vi "FindDivDigitTwoBy.vi"(0 "Normalized A":T1, 1 "premultiplied array":cluster{"A":T1, "stop":bool}[](array[cluster]), 2 "Denom Info":cluster{"Denom":i32, "Offset":i32}) -> (3 "A Copy":T1, 4 "Exact Divide":bool, 5 "Digit":i32, 6 "premultiplied array out":cluster{"A":T1, "stop":bool}[](array[cluster]))   [LabVIEW 2025]
uses:
  Number.ctl
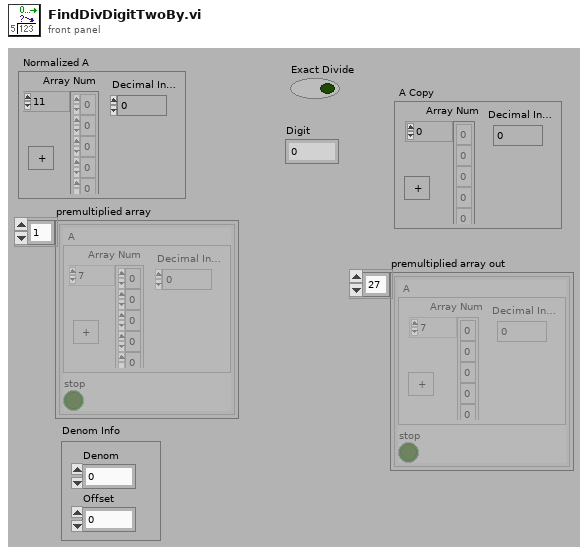
[diagram p1: front panel]
types:
  T1 = typedef "Number.ctl" = cluster{"Array Num":i8[], "Decimal Index":i32, "stop":bool}
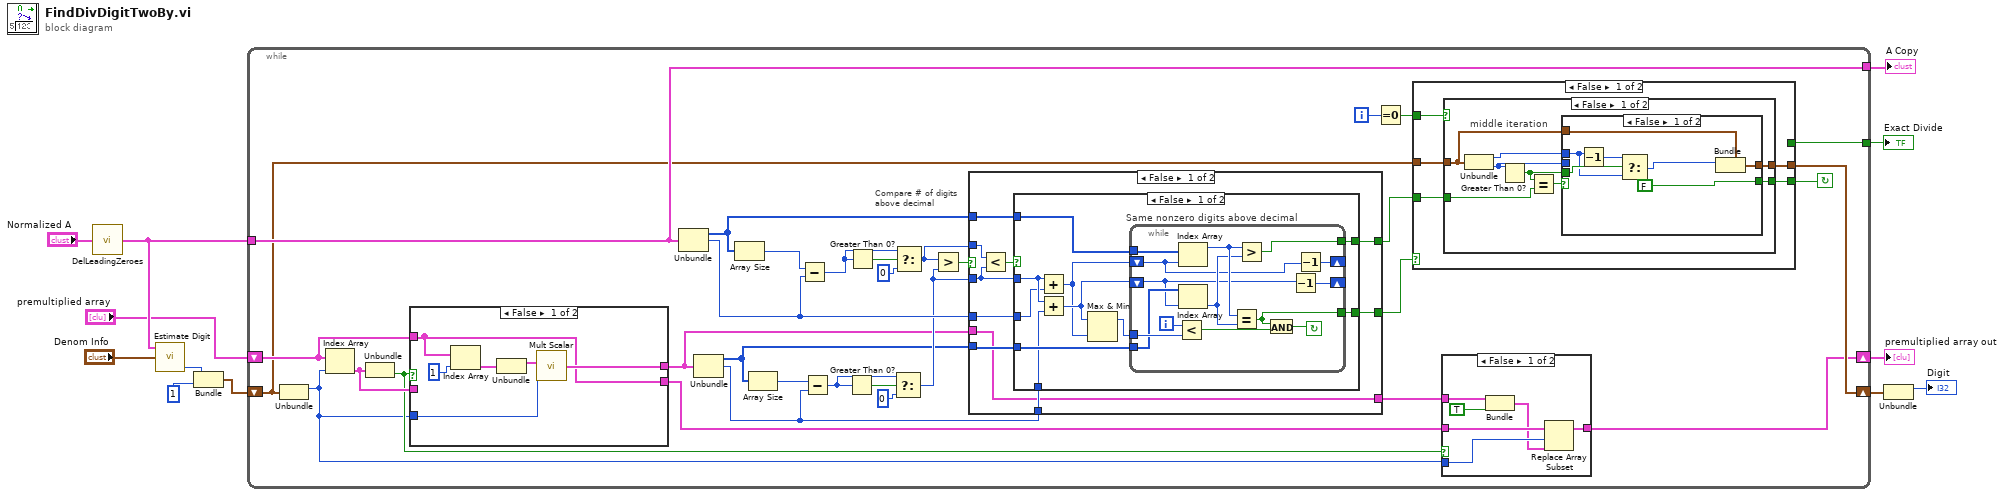
[diagram p0: block diagram]
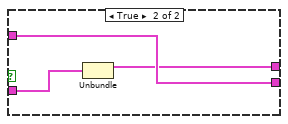
[diagram p3: hidden frame]
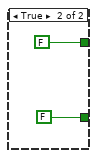
[diagram p4: hidden frame]
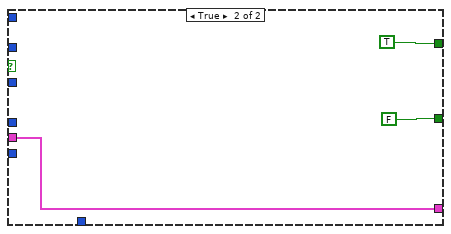
[diagram p5: hidden frame]
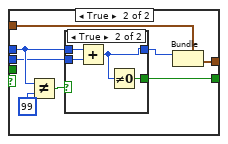
[diagram p6: hidden frame]
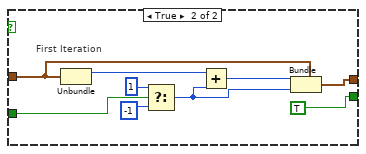
[diagram p8: hidden frame]
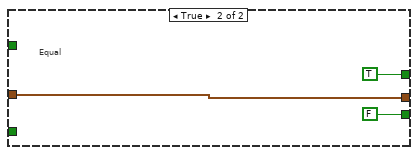
[diagram p9: hidden frame]
diagram:
  n1 = call "DelLeadingZeroes.vi"("A 2"="Normalized A") -> ("A"=w6:T1)
  n2 = call "Estimate Digit.vi"("Denom Info"="Denom Info", "A"=w6) -> ("Estimated Digit"=w5:i32)  [unwired: 3 in]
  n3 = Bundle("Estimated Digit"=w5, 1) -> (w3:cluster{"Estimated Digit":i32, i32})  [unwired: 1 in]
  n4 = while {
    tunnel: w6 -> [w24]
    shift-right: [w44] -> w10
    shift-left: w3 -> [w22]
    tunnel: [w42] -> w12
    tunnel: [w24] -> w8
    shift-right: [w19] -> w7
    shift-left: "premultiplied array" -> [w23]
    i -> [w13]
    stop <- w43 continue-if-true
    # "Compare # of digits above decimal"
    n5 = Unbundle(w22) -> ("Estimated Digit"=w17:i32)  [unwired: 1 out]
    n6 = Index Array(array=w23, index=w17) -> (element=w21:cluster{"A":T1, "stop":bool})
    n7 = Unbundle(w21) -> ("stop"=w18:bool)  [unwired: 1 out]
    n8 = case shown="False" w18 {
      tunnel: [w55 w58] -> w16
      tunnel: w17 -> [w57 _]
      tunnel: w23 -> [w52 w60]
      tunnel: [w52 w60] -> w20
      tunnel: w21 -> [_ w59]
      frame False {
        n9 = Index Array(array=w52, index=1 ("f")) -> (element=w53:cluster{"A":T1, "stop":bool})
        n10 = Unbundle(w53) -> ("A"=w56:T1)  [unwired: 1 out]
        n11 = call "Mult Scalar.vi"("A"=w56, "Scalar"=w57) -> ("A x Scalar"=w55:T1)  [unwired: 3 in]
      }
      frame True {
        n12 = Unbundle(w59) -> ("A"=w58:T1)  [unwired: 1 out]
      }
    }
    n13 = Unbundle(w24) -> ("Array Num"=w27:i8[], "Decimal Index"=w40:i32)  [unwired: 1 out]
    n14 = Unbundle(w16) -> ("Array Num"=w29:i8[], "Decimal Index"=w39:i32)  [unwired: 1 out]
    n15 = Array Size(array=w27) -> (size(s)=w28:i32)
    n16 = Array Size(array=w29) -> (size(s)=w30:i32)
    n17 = Subtract(x=w28, y=w40) -> (x-y=w32:i32)
    n18 = Subtract(x=w30, y=w39) -> (x-y=w31:i32)
    n19 = Greater Than 0?(x=w31) -> (x > 0?=w35:bool)
    n20 = Greater Than 0?(x=w32) -> (x > 0?=w36:bool)
    n21 = Select(t=w31, s=w35, f=0) -> (s? t:f=w33:i32)
    n22 = Select(t=w32, s=w36, f=0) -> (s? t:f=w37:i32)
    n23 = Greater?(x=w37, y=w33) -> (0:w41:bool)
    n24 = case shown="False" w41 {
      tunnel: [w69 TRUE] -> w26
      tunnel: w29 -> [w68 _]
      tunnel: w33 -> [w63 _]
      tunnel: w37 -> [w62 _]
      tunnel: w27 -> [w67 _]
      tunnel: [w66 FALSE] -> w25
      tunnel: w40 -> [w65 _]
      tunnel: w39 -> [w64 _]
      tunnel: w16 -> [w61 w97]
      tunnel: [w61 w97] -> w15
      frame False {
        n25 = Less?(x=w62, y=w63) -> (x < y?=w70:bool)
        n26 = case shown="False" w70 {
          tunnel: [w78 FALSE] -> w69
          tunnel: w68 -> [w79 _]
          tunnel: w67 -> [w80 _]
          tunnel: [w74 FALSE] -> w66
          tunnel: w65 -> [w76 _]
          tunnel: w64 -> [w75 _]
          tunnel: w63 -> [w77 _]
          frame False {
            # "Same nonzero digits above decimal"
            n27 = Add(x=w77, y=w76) -> (x+y=w71:i32)
            n28 = Add(x=w77, y=w75) -> (x+y=w72:i32)
            n29 = Max & Min(x=w72, y=w71) -> (max(x,y)=w73:i32)  [unwired: 1 out]
            n30 = while {
              tunnel: w73 -> [w88]
              tunnel: [w89] -> w74
              tunnel: [w90] -> w78
              tunnel: w79 -> [w85]
              tunnel: w80 -> [w86]
              shift-right: [w83] -> _
              shift-left: w71 -> [w81]
              shift-right: [w84] -> _
              shift-left: w72 -> [w82]
              i -> [w87]
              stop <- w93 continue-if-true
              n31 = Less?(x=w87, y=w88) -> (x < y?=w94:bool)
              n32 = Index Array(array=w86, index=w81) -> (element=w92:i8)
              n33 = Index Array(array=w85, index=w82) -> (element=w91:i8)
              n34 = Equal?(x=w92, y=w91) -> (x = y?=w89:bool)
              n35 = Greater?(x=w92, y=w91) -> (0:w90:bool)
              n36 = And(x=w89, y=w94) -> (x .and. y?=w93:bool)
              n37 = Decrement(x=w82) -> (x-1=w84:i32)
              n38 = Decrement(x=w81) -> (x-1=w83:i32)
            }
          }
          frame True {
          }
        }
      }
      frame True {
      }
    }
    n39 = Equal To 0?(x=w13) -> (x = 0?=w14:bool)
    n40 = case shown="False" w25 {
      tunnel: w22 -> [w102 w145]
      tunnel: w26 -> [w103 _]
      tunnel: w14 -> [w104 _]
      tunnel: [w101 w145] -> w44
      tunnel: [w100 FALSE] -> w43
      tunnel: [_ TRUE] -> w42
      frame False {
        n41 = case shown="False" w104 {
          tunnel: w103 -> [w112 w142]
          tunnel: w102 -> [w106 w137]
          tunnel: [w109 w135] -> w101
          tunnel: [w110 TRUE] -> w100
          frame False {
            # "middle iteration"
            n42 = Unbundle(w106) -> ("Estimated Digit"=w107:i32, w108:i32)
            n43 = Greater Than 0?(x=w108) -> (x > 0?=w105:bool)
            n44 = Equal?(x=w105, y=w112) -> (x = y?=w111:bool)
            n45 = case shown="False" w111 {
              tunnel: [FALSE w120] -> w110
              tunnel: [w115 w127] -> w109
              tunnel: w108 -> [_ w122]
              tunnel: w107 -> [w117 w123]
              tunnel: w106 -> [w113 w126]
              tunnel: w105 -> [w118 _]
              frame False {
                n46 = Decrement(x=w117) -> (x-1=w116:i32)
                n47 = Select(t=w116, s=w118, f=w117) -> (s? t:f=w114:i32)
                n48 = Bundle(cluster=w113, "Estimated Digit"=w114) -> (w115:cluster{"Estimated Digit":i32, i32})  [unwired: 1 in]
              }
              frame True {
                n49 = Not Equal?(x=w123, y=99) -> (x != y?=w124:bool)
                n50 = case shown="True" w124 {
                  selector: w124 -> [w128 _]
                  tunnel: w123 -> [w129 w133]
                  tunnel: w122 -> [_ w132]
                  tunnel: [w129 w131] -> w121
                  tunnel: [w128 w130] -> w120
                  frame False {
                  }
                  frame True {
                    n51 = Add(x=w133, y=w132) -> (x+y=w131:i32)
                    n52 = Not Equal To 0?(x=w131) -> (x != 0?=w130:bool)
                  }
                }
                n53 = Bundle(cluster=w126, "Estimated Digit"=w121) -> (w127:cluster{"Estimated Digit":i32, i32})  [unwired: 1 in]
              }
            }
          }
          frame True {
            # "First Iteration"
            n54 = Unbundle(w137) -> ("Estimated Digit"=w138:i32)  [unwired: 1 out]
            n55 = Select(t=1, s=w142, f=-1) -> (s? t:f=w136:i32)
            n56 = Add(x=w138, y=w136) -> (x+y=w139:i32)
            n57 = Bundle(cluster=w137, "Estimated Digit"=w139, w136) -> (w135:cluster{"Estimated Digit":i32, i32})
          }
        }
      }
      frame True {
        # "Equal"
      }
    }
    n58 = case shown="False" w18 {
      tunnel: w20 -> [w50 w51]
      tunnel: [w49 w51] -> w19
      tunnel: w17 -> [w48 _]
      tunnel: w15 -> [w47 _]
      frame False {
        n59 = Bundle("A"=w47, TRUE) -> (w45:cluster{"A":T1, bool})  [unwired: 1 in]
        n60 = Replace Array Subset(array=w50, new element=w45, index=w48) -> (w49:cluster{"A":T1, "stop":bool}[])
      }
      frame True {
      }
    }
  }
  "Exact Divide" <- w12
  "A Copy" <- w8
  "premultiplied array out" <- w7
  n61 = Unbundle(w10) -> ("Estimated Digit"=→"Digit":i32)  [unwired: 1 out]
